vi "ramp.vi"(8 "start":i32, 11 "end":i32) -> (3 "ramp":dbl[](array[numeric]))   [LabVIEW 2014, in "NI_AALPro.lvlib"]
uses:
  NI_AALPro.lvlib
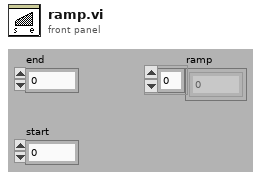
[diagram p1: front panel]
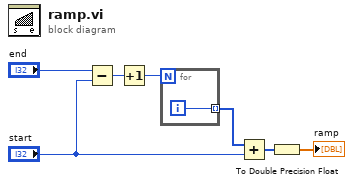
[diagram p0: block diagram]
diagram:
  n1 = Subtract(x="end", y="start") -> (x-y=w6:i32)
  n2 = Increment(x=w6) -> (x+1=w5:i32)
  n3 = for {
    N: w5 -> [_]
    tunnel: [w8] -> w4 mode=indexing
    i -> [w8]
  }
  n4 = Add(x=w4, y="start") -> (x+y=w2:i32[])
  n5 = To Double Precision Float(number=w2) -> (double precision float=→"ramp":dbl[])
